vi "fpga_LineInputs-Conn2-Set2.vi"() -> (0 "DataLines":T1)   [LabVIEW 2011]
uses:
  <vilib>/rvi/eio/common/nirviEmuTemplateMethod_errors.vi
  <vilib>/eio/EIONode/EIONode.xnode
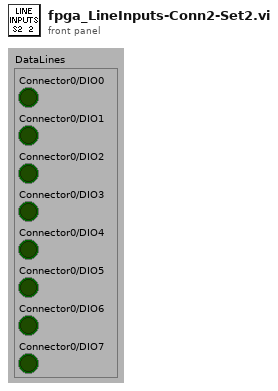
[diagram p1: front panel]
types:
  T1 = cluster{"Connector0/DIO0":bool, "Connector0/DIO1":bool, "Connector0/DIO2":bool, "Connector0/DIO3":bool, "Connector0/DIO4":bool, "Connector0/DIO5":bool, "Connector0/DIO6":bool, "Connector0/DIO7":bool}
  T2 = cluster{"Connector2/DIO16":bool, "Connector2/DIO17":bool, "Connector2/DIO18":bool, "Connector2/DIO19":bool, "Connector2/DIO20":bool, "Connector2/DIO21":bool, "Connector2/DIO22":bool, "Connector2/DIO23":bool}
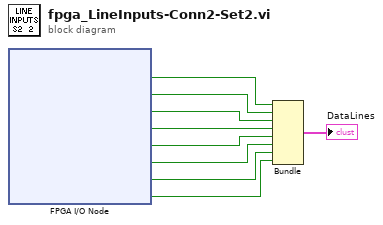
[diagram p0: block diagram]
diagram:
  n1 = xnode "FPGA I/O Node"() -> ("Connector2/DIO16"=w9:bool, "Connector2/DIO17"=w8:bool, "Connector2/DIO18"=w7:bool, "Connector2/DIO19"=w6:bool, "Connector2/DIO20"=w5:bool, "Connector2/DIO21"=w4:bool, "Connector2/DIO22"=w3:bool, "Connector2/DIO23"=w2:bool)  [unwired: 8 in, 8 out]
  n2 = Bundle("Connector2/DIO16"=w9, "Connector2/DIO17"=w8, "Connector2/DIO18"=w7, "Connector2/DIO19"=w6, "Connector2/DIO20"=w5, "Connector2/DIO21"=w4, "Connector2/DIO22"=w3, "Connector2/DIO23"=w2) -> (→"DataLines":T2)  [unwired: 1 in]
